vi "Post Build Script.vi"(0 "PostBuildSupport in":refnum<class "PostBuildSupport.lvclass">, 5 "error in (no error)":errorcluster) -> (19 "error out":errorcluster)   [LabVIEW 2016, in "PostBuildSupport.lvclass"]
uses:
  PostBuildSupport.lvclass
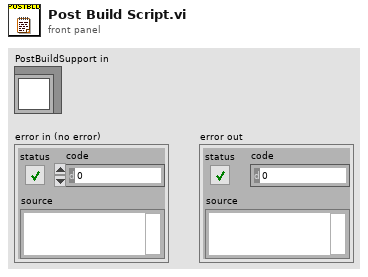
[diagram p1: front panel]
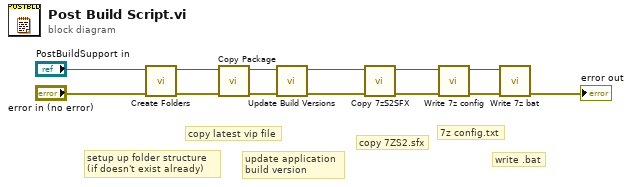
[diagram p0: block diagram]
diagram:
  # "copy 7ZS2.sfx"
  # "setup up folder structure \n(if doesn't exist already)"
  # "update application\nbuild version"
  # "copy latest vip file"
  # "7z config.txt"
  # "write .bat"
  n1 = call "Create Folders.vi"("error in (no error)"="error in (no error)", "PostBuildSupport in"="PostBuildSupport in") -> ("error out"=w1:errorcluster, "PostBuildSupport out"=w2:refnum<class "PostBuildSupport.lvclass">)  [unwired: 8 in]
  n2 = call "Copy Package.vi"("error in (no error)"=w1, "PostBuildSupport in"=w2) -> ("error out"=w9:errorcluster, "PostBuildSupport out"=w10:refnum<class "PostBuildSupport.lvclass">)  [unwired: 8 in]
  n3 = call "Update Build Versions.vi"("error in (no error)"=w9, "PostBuildSupport in"=w10) -> ("error out"=w6:errorcluster, "PostBuildSupport out"=w4:refnum<class "PostBuildSupport.lvclass">)  [unwired: 8 in]
  n4 = call "Copy 7zS2SFX.vi"("error in (no error)"=w6, "PostBuildSupport in"=w4) -> ("error out"=w5:errorcluster, "PostBuildSupport out"=w3:refnum<class "PostBuildSupport.lvclass">)  [unwired: 8 in]
  n5 = call "Write 7z config.vi"("error in (no error)"=w5, "PostBuildSupport in"=w3) -> ("error out"=w8:errorcluster, "PostBuildSupport out"=w11:refnum<class "PostBuildSupport.lvclass">)  [unwired: 8 in]
  n6 = call "Write 7z bat.vi"("error in (no error)"=w8, "PostBuildSupport in"=w11) -> ("error out"=→"error out":errorcluster)  [unwired: 8 in, 1 out]
